vi "_Enqueue JKISMQ.vi"(8 "Error in":errorcluster caption="Error in (no error)", 10 "Data":T1, 11 "JKISMQ":T2) -> (0 "Error out":errorcluster, 1 "Target Buzy Error":bool, 3 "JKISMQ":T2)   [LabVIEW 2020, in "JKI-State-Machine-Plus.lvlib"]
uses:
  JKI-State-Machine-Plus.lvlib
  _JKISMQ.ctl
  _Cross JKI StateMachine State Data.ctl
  _Cross JKI StateMachine State Response.ctl
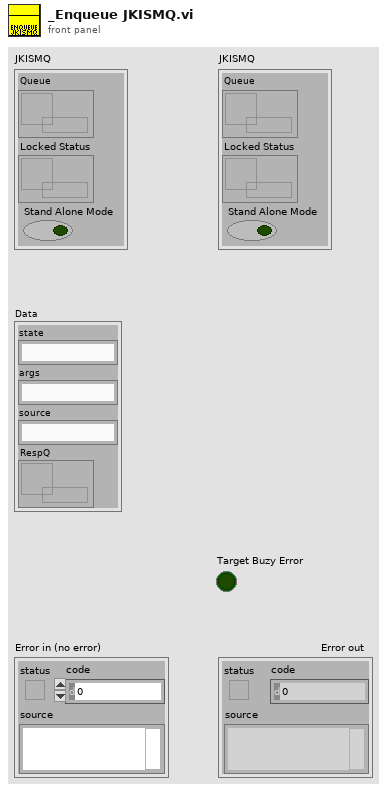
[diagram p1: front panel]
types:
  T1 = typedef "JKI-State-Machine-Plus.lvlib/_Cross JKI StateMachine State Data.ctl" = cluster{"state":string, "args":string, "source":string, "RespQ":refnum<queue>}
  T2 = typedef "JKI-State-Machine-Plus.lvlib/_JKISMQ.ctl" = cluster{"Queue":refnum<queue>, "Locked Status":refnum<data-value>, "Stand Alone Mode":bool}
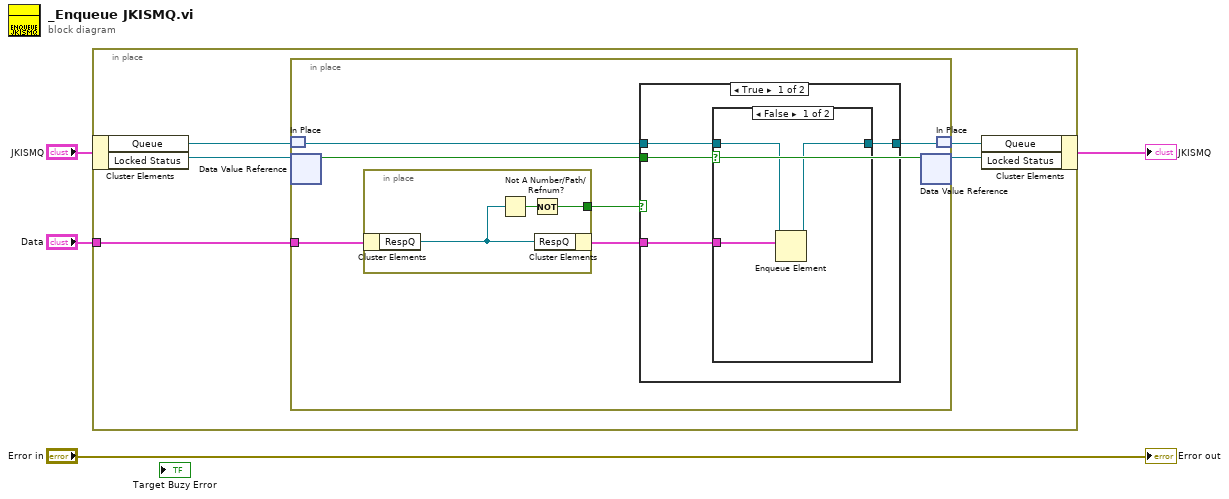
[diagram p0: block diagram]
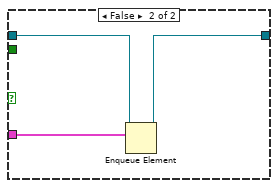
[diagram p3: hidden frame]
diagram:
  n1 = in-place "In Place Element Structure" {
    in-place-border: "Data" -> [w5]
    n2 = in-place-cluster #1("JKISMQ") -> ("Queue"=w9:refnum<queue>, "Locked Status"=w7:refnum<data-value>)
    n3 = in-place {
      in-place-border: w5 -> [w13]
      n4 = in-place-match #2(w9) -> (w14:refnum<queue>)
      n5 = in-place-dvr #3(w7) -> (w10:bool)  [unwired: 1 out]
      n6 = in-place {
        in-place-border: [w27] -> w11
        n7 = in-place-cluster #4(w13) -> ("RespQ"=w29:refnum<queue>)
        n8 = Not A Number/Path/Refnum?(number/path/refnum=w29) -> (NaN/Path/Refnum?=w28:bool)
        n9 = Not(x=w28) -> (.not. x?=w27:bool)
        n10 = in-place-cluster #4("RespQ"=w29) -> (w12:T1)
      }
      n11 = case shown="True" w11 {
        tunnel: [w19 w26] -> w15
        tunnel: w14 -> [w18 w25]
        tunnel: w12 -> [w17 w24]
        tunnel: w10 -> [w16 _]
        frame True {
          n12 = case shown="False" w16 {
            tunnel: [w22 w23] -> w19
            tunnel: w18 -> [w21 w23]
            tunnel: w17 -> [w20 _]
            frame False {
              n13 = Enqueue Element(queue=w21, element=w20) -> (queue out=w22:refnum<queue>)  [unwired: 2 in, 2 out]
            }
            frame True {
            }
          }
        }
        frame False {
          n14 = Enqueue Element(queue=w25, element=w24) -> (queue out=w26:refnum<queue>)  [unwired: 2 in, 2 out]
        }
      }
      n15 = in-place-dvr #3(w10) -> (w6:refnum<data-value>)  [unwired: 1 out]
      n16 = in-place-match #2(w15) -> (w8:refnum<queue>)
    }
    n17 = in-place-cluster #1("Queue"=w8, "Locked Status"=w6) -> (→"JKISMQ":T2)
  }
  "Error out" <- "Error in"
